vi "LeastSquareCalculation.vi"(6 "array 4":dbl[](array[numeric]), 9 "array 3":dbl[](array[numeric]), 10 "array 2":dbl[](array[numeric]), 11 "array":dbl[](array[numeric])) -> (3 "Numeric":dbl)   [LabVIEW 2013]
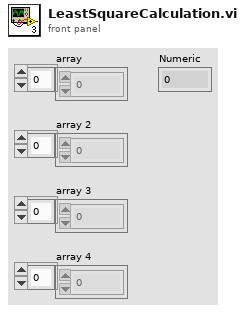
[diagram p1: front panel]
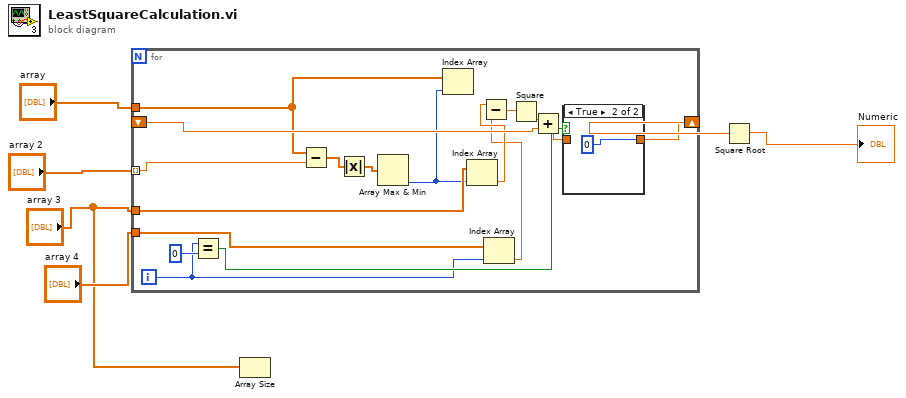
[diagram p0: block diagram]
diagram:
  n1 = for {
    tunnel: "array 2" -> [w18] mode=indexing
    shift-right: [w14] -> w3
    shift-left: _ -> [w19]
    tunnel: "array" -> [w17]
    tunnel: "array 4" -> [w12]
    tunnel: "array 3" -> [w11]
    i -> [w7]
    n2 = Equal?(x=w7, y=0) -> (x = y?=w15:bool)
    n3 = Subtract(x=w17, y=w18) -> (x-y=w23:dbl[])
    n4 = Absolute Value(x=w23) -> (abs(x)=w22:dbl[])
    n5 = Array Max & Min(array=w22) -> (min index (indices)=w10:i32)  [unwired: 3 out]
    n6 = Index Array(array=w17, index=w10) -> ()  [unwired: 1 out]
    n7 = Index Array(array=w11, index=w10) -> (element=w9:dbl)
    n8 = Index Array(array=w12, index=w7) -> (element=w8:dbl)
    n9 = Subtract(x=w9, y=w8) -> (x-y=w21:dbl)
    n10 = Square(x=w21) -> (x^2=w20:dbl)
    n11 = Add(x=w20, y=w19) -> (x+y=w13:dbl)
    n12 = case shown="True" w15 {
      tunnel: [w24 0 ("y")] -> w14
      tunnel: w13 -> [w24 _]
      frame False {
      }
      frame True {
      }
    }
  }
  n13 = Array Size(array="array 3") -> ()  [unwired: 1 out]
  n14 = Square Root(x=w3) -> (sqrt(x)=→"Numeric":dbl)
